vi "LaserControl.vi"() -> ()   [LabVIEW 2015]
uses:
  <vilib>/DAQmx/write.llb/DAQmx Write (Digital Bool 1Line 1Point).vi
  <vilib>/DAQmx/write.llb/DAQmx Write (Analog DBL 1Chan 1Samp).vi
  <vilib>/DAQmx/write.llb/DAQmx Write (Digital 1D Bool NChan 1Samp 1Line).vi
  <vilib>/DAQmx/create/channels.llb/DAQmx Create Channel (DO-Digital Output).vi
  <vilib>/DAQmx/miscellaneous.llb/DAQmx Fill In Error Info.vi
  <vilib>/DAQmx/create/channels.llb/DAQmx Create Channel (AO-Voltage-Basic).vi
panel:
  in  "blueV":dbl
  in  "greenV":dbl
  in  "redV":dbl
  in  "blueAO":dbl(slide) min=0.0 max=5.0 step=0.001 scale=0.0..5.0
  in  "greenAO":dbl(slide) min=0.0 max=5.0 step=0.001 scale=0.0..5.0
  in  "ChangeAOM":bool
  in  "OK Button":bool
  in  "all off":bool
  in  "redAO":dbl(slide) min=0.0 max=5.0 step=0.0001 scale=0.0..5.0
  in  "Green Laser":bool
  in  "Blue Laser":bool
  in  "Red Laser":bool
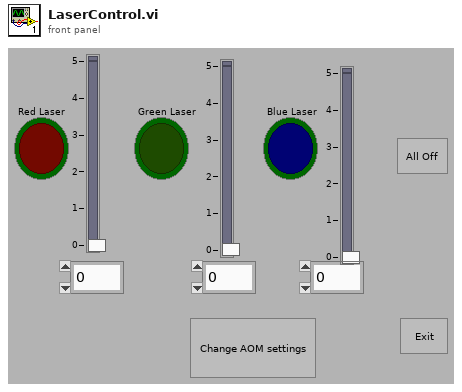
[diagram p1: front panel]
types:
  T1 = typedef "XYZStage.lvlib/XYZStage Configuration.ctl" = cluster{"VISA resource name":refnum<visa-resource-name>, "Timeout (3sec)":u32}
  T2 = cluster{"StageS":i32, "StageL":i32, "currmeas data dir":path, "image OD":u16, "contour OD":u16, "point OD":u16, "AOlines":tag[], "AIlines":tag[], "CI lines":tag[], "DO lines":tag[], "AO names":string[], "CI names":string[], "AI names":string[], "DO names":string[], "CIextensions":string[], "AIextensions":string[], "Voltage to Ygalvo":i32, "Voltage to Xgalvo":i32, "Voltage to patch":i32, "640 shutter":i32, "2P shutter":i32, "LT timestamp":u32, "Vp":i32, "Ip":i32, "camera trigger":i32, "master data dir":path, "voltage to Zpos":i32, "Vto2P":i32, "640 AO":i32, "488 AO":i32, "532 AO":i32, "640TTL":u32, "488TTL":u32, "532TTL":u32, "Device 1 sampleclock out":tag, "Device 1 Starttrigger out":tag, "Device 2 sampleclock in":tag, "Device 2 StartTrigger in ":tag, "2PODTTL":u32, "488 shutter":u32, "LCVR red":u32, "LCVR blue":u32, "Sutter Stage Config":T1}
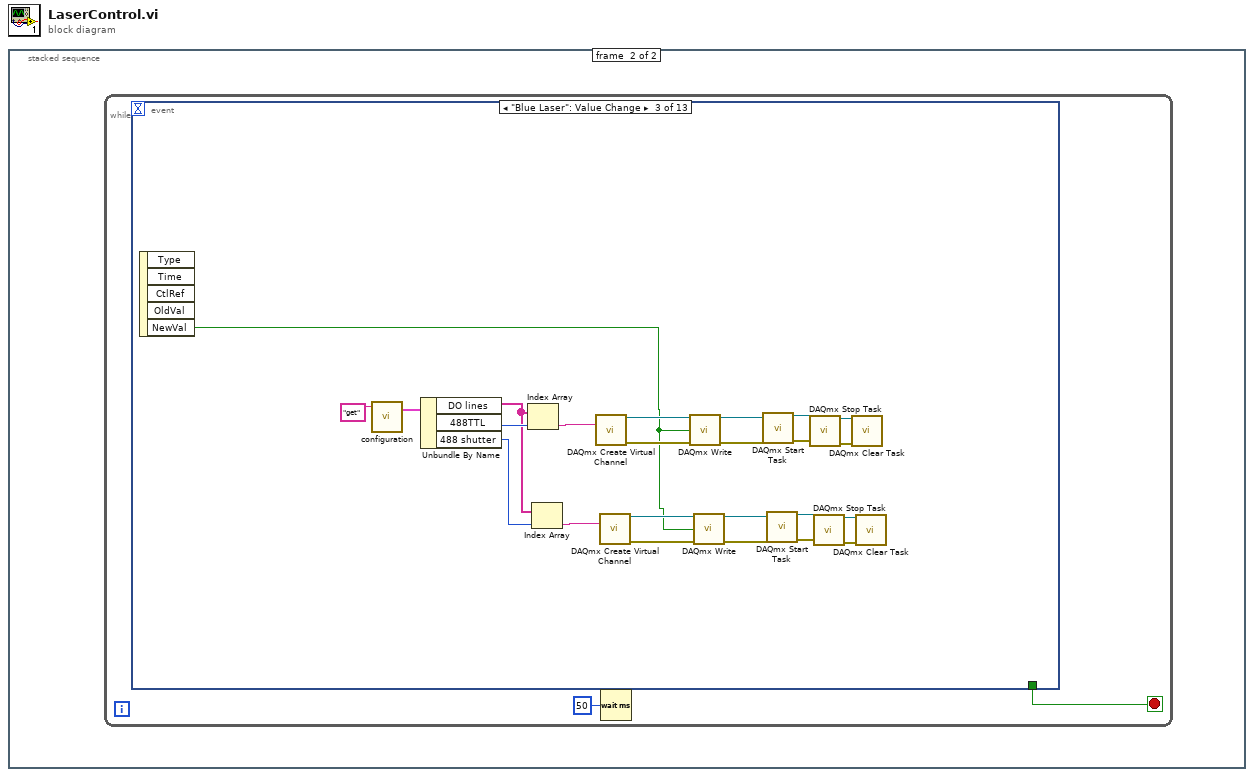
[diagram p0: block diagram]
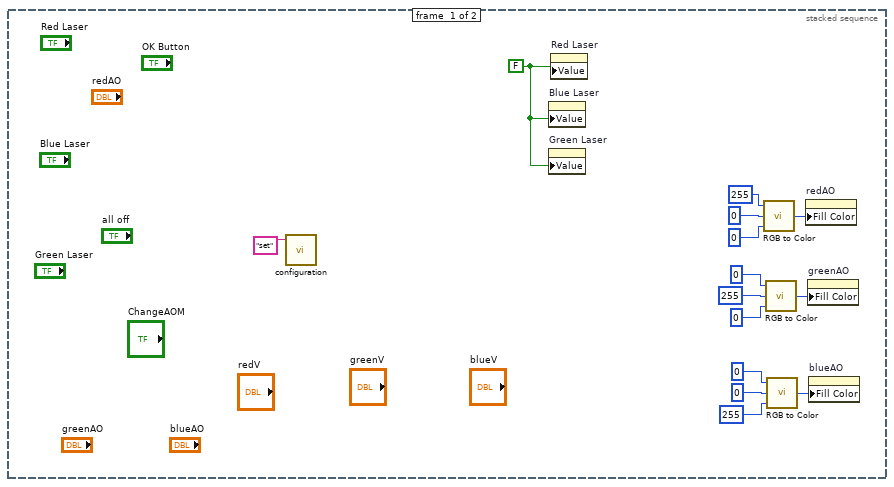
[diagram p2: hidden frame]
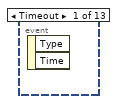
[diagram p3: hidden frame]
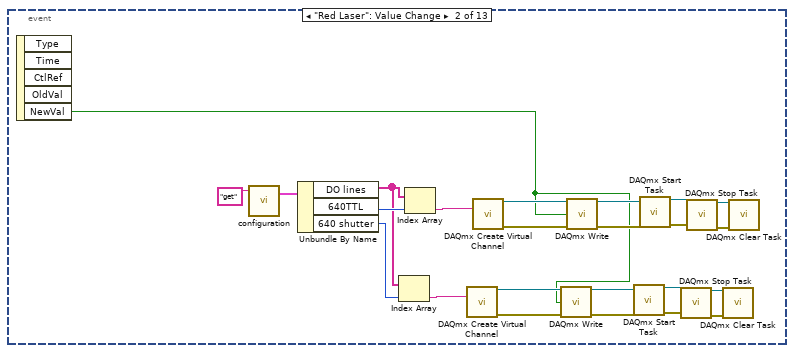
[diagram p4: hidden frame]
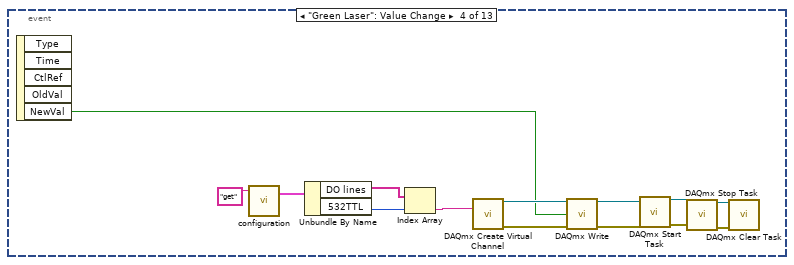
[diagram p5: hidden frame]
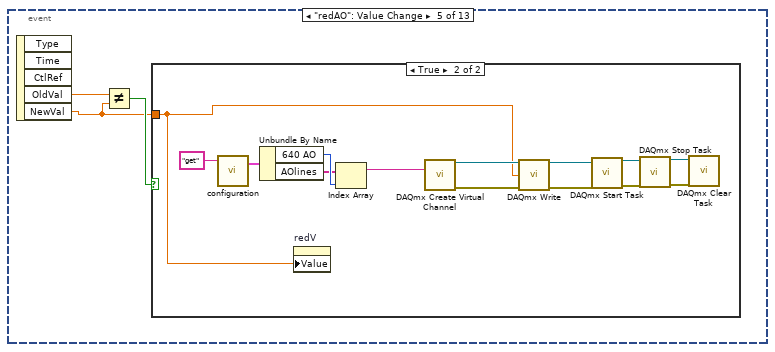
[diagram p6: hidden frame]
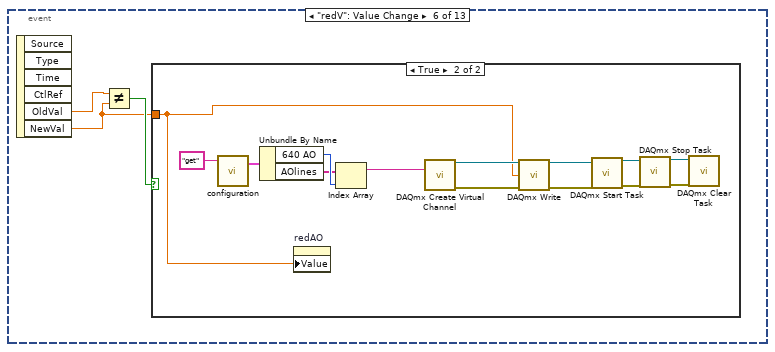
[diagram p8: hidden frame]
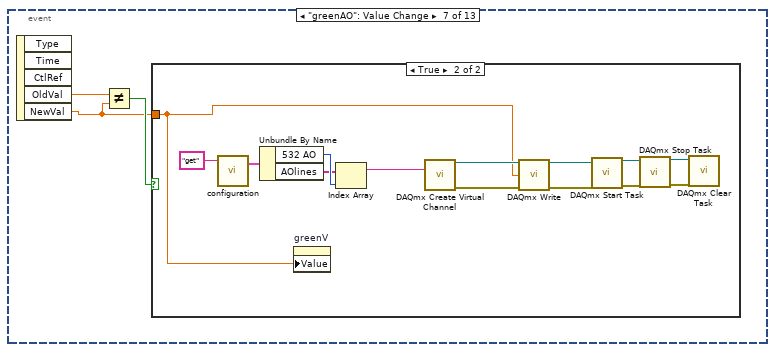
[diagram p10: hidden frame]
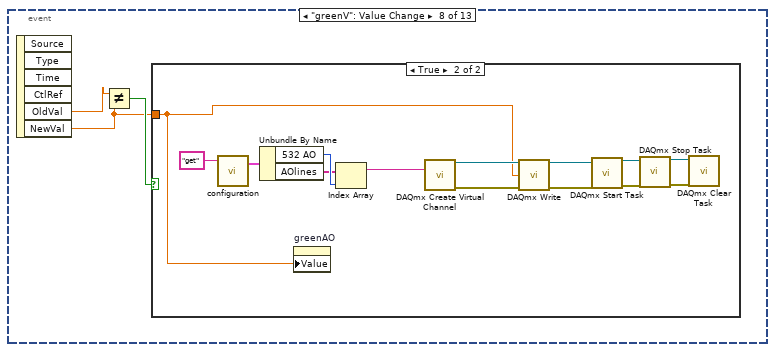
[diagram p12: hidden frame]
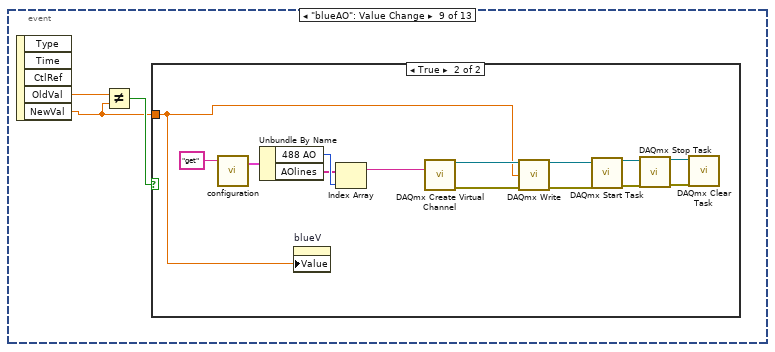
[diagram p14: hidden frame]
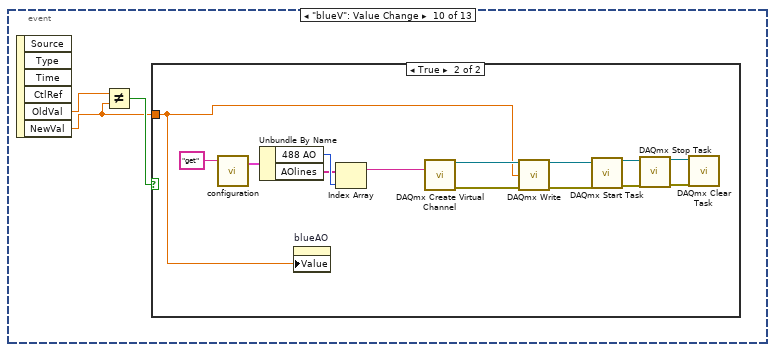
[diagram p16: hidden frame]
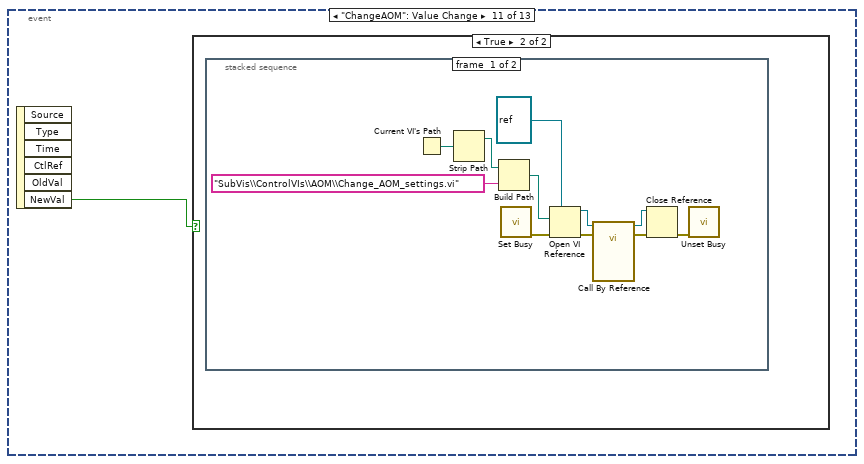
[diagram p18: hidden frame]
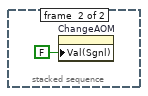
[diagram p20: hidden frame]
diagram:
  n1 = stacked-sequence {
    frame #0 {
      w13 = FALSE
      n2 = call "configuration.vi"("command"="set") -> ()  [unwired: 2 in, 2 out]
      n3 = property on="Blue Laser" class="Bool (strict)"("Value"=w13) -> ()  [unwired: 2 in, 2 out]
      n4 = property on="Green Laser" class="Bool (strict)"("Value"=w13) -> ()  [unwired: 2 in, 2 out]
      n5 = property on="Red Laser" class="Bool (strict)"("Value"=w13) -> ()  [unwired: 2 in, 2 out]
      n6 = call <vilib>:"RGB to Color.vi"("B"=u8 0, "G"=u8 0, "R"=255) -> ("Color"=w14:u32)
      n7 = call <vilib>:"RGB to Color.vi"("B"=u8 0, "G"=u8 255, "R"=0) -> ("Color"=w5:u32)
      n8 = call <vilib>:"RGB to Color.vi"("B"=u8 255, "G"=u8 0, "R"=0) -> ("Color"=w4:u32)
      n9 = property on="redAO" class="Slide (strict)"("Fill Color"=w14) -> ()  [unwired: 2 in, 2 out]
      n10 = property on="greenAO" class="Slide (strict)"("Fill Color"=w5) -> ()  [unwired: 2 in, 2 out]
      n11 = property on="blueAO" class="Slide (strict)"("Fill Color"=w4) -> ()  [unwired: 2 in, 2 out]
    }
    frame #1 {
      n12 = while {
        stop <- w16 stop-if-true
        n13 = event shown="[2] \"Blue Laser\": Value Change" {
          selector: _ -> [_ _ _ _ _ _ _ _ _ _ _ _ _]
          dyn-events: _ -> [_ _ _ _ _ _ _ _ _ _ _ _ _]
          timeout: _ -> [_ _ _ _ _ _ _ _ _ _ _ _ _]
          tunnel: [_ _ _ _ _ _ _ _ _ _ _ _ w220] -> w16
          event Timeout {
            n14 = event-data() -> ()  [unwired: 1 in, 2 out]
          }
          event "Red Laser": Value Change {
            n15 = event-data() -> ("NewVal"=w17:bool)  [unwired: 1 in, 4 out]
            n16 = call "configuration.vi"("command"="get") -> ("config out"=w31:T2)  [unwired: 2 in, 1 out]
            n17 = Unbundle By Name(w31) -> ("DO lines"=w18:tag[], "640TTL"=w30:u32, "640 shutter"=w19:i32)
            n18 = Index Array(array=w18, index=w19) -> (element=w28:tag)
            n19 = Index Array(array=w18, index=w30) -> (element=w29:tag)
            n20 = call-poly <vilib>:"DAQmx Create Virtual Channel.vi"("lines"=w28) -> ("task out"=w26:refnum<k21>, "error out"=w27:errorcluster)  [unwired: 13 in]
            n21 = call-poly <vilib>:"DAQmx Create Virtual Channel.vi"("lines"=w29) -> ("task out"=w34:refnum<k21>, "error out"=w33:errorcluster)  [unwired: 13 in]
            n22 = call-poly <vilib>:"DAQmx Write.vi"("task/channels in"=w26, "data"=w17, "error in"=w27) -> ("task out"=w25:refnum<k21>, "error out"=w24:errorcluster)  [unwired: 10 in, 1 out]
            n23 = call-poly <vilib>:"DAQmx Write.vi"("task/channels in"=w34, "data"=w17, "error in"=w33) -> ("task out"=w35:refnum<k21>, "error out"=w36:errorcluster)  [unwired: 10 in, 1 out]
            n24 = call <vilib>:"DAQmx Start Task.vi"("task/channels in"=w25, "error in"=w24) -> ("task out"=w23:refnum<k21>, "error out"=w22:errorcluster)  [unwired: 12 in]
            n25 = call <vilib>:"DAQmx Start Task.vi"("task/channels in"=w35, "error in"=w36) -> ("task out"=w37:refnum<k21>, "error out"=w38:errorcluster)  [unwired: 12 in]
            n26 = call <vilib>:"DAQmx Stop Task.vi"("task/channels in"=w23, "error in"=w22) -> ("task out"=w21:refnum<k21>, "error out"=w20:errorcluster)  [unwired: 12 in]
            n27 = call <vilib>:"DAQmx Stop Task.vi"("task/channels in"=w37, "error in"=w38) -> ("task out"=w39:refnum<k21>, "error out"=w40:errorcluster)  [unwired: 12 in]
            n28 = call <vilib>:"DAQmx Clear Task.vi"("task in"=w21, "error in"=w20) -> ()  [unwired: 13 in, 1 out]
            n29 = call <vilib>:"DAQmx Clear Task.vi"("task in"=w39, "error in"=w40) -> ()  [unwired: 13 in, 1 out]
          }
          event "Blue Laser": Value Change {
            n30 = event-data() -> ("NewVal"=w43:bool)  [unwired: 1 in, 4 out]
            n31 = call "configuration.vi"("command"="get") -> ("config out"=w55:T2)  [unwired: 2 in, 1 out]
            n32 = Unbundle By Name(w55) -> ("DO lines"=w42:tag[], "488TTL"=w54:u32, "488 shutter"=w41:u32)
            n33 = Index Array(array=w42, index=w54) -> (element=w53:tag)
            n34 = Index Array(array=w42, index=w41) -> (element=w52:tag)
            n35 = call-poly <vilib>:"DAQmx Create Virtual Channel.vi"("lines"=w53) -> ("task out"=w58:refnum<k21>, "error out"=w57:errorcluster)  [unwired: 13 in]
            n36 = call-poly <vilib>:"DAQmx Create Virtual Channel.vi"("lines"=w52) -> ("task out"=w50:refnum<k21>, "error out"=w51:errorcluster)  [unwired: 13 in]
            n37 = call-poly <vilib>:"DAQmx Write.vi"("task/channels in"=w58, "data"=w43, "error in"=w57) -> ("task out"=w59:refnum<k21>, "error out"=w60:errorcluster)  [unwired: 10 in, 1 out]
            n38 = call-poly <vilib>:"DAQmx Write.vi"("task/channels in"=w50, "data"=w43, "error in"=w51) -> ("task out"=w49:refnum<k21>, "error out"=w48:errorcluster)  [unwired: 10 in, 1 out]
            n39 = call <vilib>:"DAQmx Start Task.vi"("task/channels in"=w59, "error in"=w60) -> ("task out"=w61:refnum<k21>, "error out"=w62:errorcluster)  [unwired: 12 in]
            n40 = call <vilib>:"DAQmx Start Task.vi"("task/channels in"=w49, "error in"=w48) -> ("task out"=w47:refnum<k21>, "error out"=w46:errorcluster)  [unwired: 12 in]
            n41 = call <vilib>:"DAQmx Stop Task.vi"("task/channels in"=w61, "error in"=w62) -> ("task out"=w63:refnum<k21>, "error out"=w64:errorcluster)  [unwired: 12 in]
            n42 = call <vilib>:"DAQmx Stop Task.vi"("task/channels in"=w47, "error in"=w46) -> ("task out"=w45:refnum<k21>, "error out"=w44:errorcluster)  [unwired: 12 in]
            n43 = call <vilib>:"DAQmx Clear Task.vi"("task in"=w63, "error in"=w64) -> ()  [unwired: 13 in, 1 out]
            n44 = call <vilib>:"DAQmx Clear Task.vi"("task in"=w45, "error in"=w44) -> ()  [unwired: 13 in, 1 out]
          }
          event "Green Laser": Value Change {
            n45 = event-data() -> ("NewVal"=w70:bool)  [unwired: 1 in, 4 out]
            n46 = call "configuration.vi"("command"="get") -> ("config out"=w68:T2)  [unwired: 2 in, 1 out]
            n47 = Unbundle By Name(w68) -> ("DO lines"=w67:tag[], "532TTL"=w66:u32)
            n48 = Index Array(array=w67, index=w66) -> (element=w65:tag)
            n49 = call-poly <vilib>:"DAQmx Create Virtual Channel.vi"("lines"=w65) -> ("task out"=w72:refnum<k21>, "error out"=w71:errorcluster)  [unwired: 13 in]
            n50 = call-poly <vilib>:"DAQmx Write.vi"("task/channels in"=w72, "data"=w70, "error in"=w71) -> ("task out"=w73:refnum<k21>, "error out"=w74:errorcluster)  [unwired: 10 in, 1 out]
            n51 = call <vilib>:"DAQmx Start Task.vi"("task/channels in"=w73, "error in"=w74) -> ("task out"=w75:refnum<k21>, "error out"=w76:errorcluster)  [unwired: 12 in]
            n52 = call <vilib>:"DAQmx Stop Task.vi"("task/channels in"=w75, "error in"=w76) -> ("task out"=w77:refnum<k21>, "error out"=w78:errorcluster)  [unwired: 12 in]
            n53 = call <vilib>:"DAQmx Clear Task.vi"("task in"=w77, "error in"=w78) -> ()  [unwired: 13 in, 1 out]
          }
          event "redAO": Value Change {
            n54 = event-data() -> ("OldVal"=w80:dbl, "NewVal"=w79:dbl)  [unwired: 1 in, 3 out]
            n55 = Not Equal?(x=w80, y=w79) -> (x != y?=w81:bool)
            n56 = case shown="True" w81 {
              tunnel: w79 -> [_ w82]
              frame False {
              }
              frame True {
                n57 = call "configuration.vi"("command"="get") -> ("config out"=w86:T2)  [unwired: 2 in, 1 out]
                n58 = Unbundle By Name(w86) -> ("640 AO"=w85:i32, "AOlines"=w84:tag[])
                n59 = property on="redV" class="DigNum (strict)"("Value"=w82) -> ()  [unwired: 2 in, 2 out]
                n60 = Index Array(array=w84, index=w85) -> (element=w83:tag)
                n61 = call-poly <vilib>:"DAQmx Create Virtual Channel.vi"("physical channels"=w83) -> ("task out"=w89:refnum<k21>, "error out"=w88:errorcluster)  [unwired: 13 in]
                n62 = call-poly <vilib>:"DAQmx Write.vi"("task/channels in"=w89, "data"=w82, "error in"=w88) -> ("task out"=w90:refnum<k21>, "error out"=w91:errorcluster)  [unwired: 10 in, 1 out]
                n63 = call <vilib>:"DAQmx Start Task.vi"("task/channels in"=w90, "error in"=w91) -> ("task out"=w92:refnum<k21>, "error out"=w93:errorcluster)  [unwired: 12 in]
                n64 = call <vilib>:"DAQmx Stop Task.vi"("task/channels in"=w92, "error in"=w93) -> ("task out"=w94:refnum<k21>, "error out"=w95:errorcluster)  [unwired: 12 in]
                n65 = call <vilib>:"DAQmx Clear Task.vi"("task in"=w94, "error in"=w95) -> ()  [unwired: 13 in, 1 out]
              }
            }
          }
          event "redV": Value Change {
            n66 = event-data() -> ("OldVal"=w97:dbl, "NewVal"=w96:dbl)  [unwired: 1 in, 4 out]
            n67 = Not Equal?(x=w97, y=w96) -> (x != y?=w98:bool)
            n68 = case shown="True" w98 {
              tunnel: w96 -> [_ w99]
              frame False {
              }
              frame True {
                n69 = call "configuration.vi"("command"="get") -> ("config out"=w103:T2)  [unwired: 2 in, 1 out]
                n70 = Unbundle By Name(w103) -> ("640 AO"=w102:i32, "AOlines"=w101:tag[])
                n71 = property on="redAO" class="Slide (strict)"("Value"=w99) -> ()  [unwired: 2 in, 2 out]
                n72 = Index Array(array=w101, index=w102) -> (element=w100:tag)
                n73 = call-poly <vilib>:"DAQmx Create Virtual Channel.vi"("physical channels"=w100) -> ("task out"=w106:refnum<k21>, "error out"=w105:errorcluster)  [unwired: 13 in]
                n74 = call-poly <vilib>:"DAQmx Write.vi"("task/channels in"=w106, "data"=w99, "error in"=w105) -> ("task out"=w107:refnum<k21>, "error out"=w108:errorcluster)  [unwired: 10 in, 1 out]
                n75 = call <vilib>:"DAQmx Start Task.vi"("task/channels in"=w107, "error in"=w108) -> ("task out"=w109:refnum<k21>, "error out"=w110:errorcluster)  [unwired: 12 in]
                n76 = call <vilib>:"DAQmx Stop Task.vi"("task/channels in"=w109, "error in"=w110) -> ("task out"=w111:refnum<k21>, "error out"=w112:errorcluster)  [unwired: 12 in]
                n77 = call <vilib>:"DAQmx Clear Task.vi"("task in"=w111, "error in"=w112) -> ()  [unwired: 13 in, 1 out]
              }
            }
          }
          event "greenAO": Value Change {
            n78 = event-data() -> ("OldVal"=w114:dbl, "NewVal"=w113:dbl)  [unwired: 1 in, 3 out]
            n79 = Not Equal?(x=w114, y=w113) -> (x != y?=w115:bool)
            n80 = case shown="True" w115 {
              tunnel: w113 -> [_ w116]
              frame False {
              }
              frame True {
                n81 = call "configuration.vi"("command"="get") -> ("config out"=w120:T2)  [unwired: 2 in, 1 out]
                n82 = Unbundle By Name(w120) -> ("532 AO"=w119:i32, "AOlines"=w118:tag[])
                n83 = property on="greenV" class="DigNum (strict)"("Value"=w116) -> ()  [unwired: 2 in, 2 out]
                n84 = Index Array(array=w118, index=w119) -> (element=w117:tag)
                n85 = call-poly <vilib>:"DAQmx Create Virtual Channel.vi"("physical channels"=w117) -> ("task out"=w123:refnum<k21>, "error out"=w122:errorcluster)  [unwired: 13 in]
                n86 = call-poly <vilib>:"DAQmx Write.vi"("task/channels in"=w123, "data"=w116, "error in"=w122) -> ("task out"=w124:refnum<k21>, "error out"=w125:errorcluster)  [unwired: 10 in, 1 out]
                n87 = call <vilib>:"DAQmx Start Task.vi"("task/channels in"=w124, "error in"=w125) -> ("task out"=w126:refnum<k21>, "error out"=w127:errorcluster)  [unwired: 12 in]
                n88 = call <vilib>:"DAQmx Stop Task.vi"("task/channels in"=w126, "error in"=w127) -> ("task out"=w128:refnum<k21>, "error out"=w129:errorcluster)  [unwired: 12 in]
                n89 = call <vilib>:"DAQmx Clear Task.vi"("task in"=w128, "error in"=w129) -> ()  [unwired: 13 in, 1 out]
              }
            }
          }
          event "greenV": Value Change {
            n90 = event-data() -> ("OldVal"=w131:dbl, "NewVal"=w130:dbl)  [unwired: 1 in, 4 out]
            n91 = Not Equal?(x=w131, y=w130) -> (x != y?=w132:bool)
            n92 = case shown="True" w132 {
              tunnel: w130 -> [_ w133]
              frame False {
              }
              frame True {
                n93 = call "configuration.vi"("command"="get") -> ("config out"=w137:T2)  [unwired: 2 in, 1 out]
                n94 = Unbundle By Name(w137) -> ("532 AO"=w136:i32, "AOlines"=w135:tag[])
                n95 = property on="greenAO" class="Slide (strict)"("Value"=w133) -> ()  [unwired: 2 in, 2 out]
                n96 = Index Array(array=w135, index=w136) -> (element=w134:tag)
                n97 = call-poly <vilib>:"DAQmx Create Virtual Channel.vi"("physical channels"=w134) -> ("task out"=w140:refnum<k21>, "error out"=w139:errorcluster)  [unwired: 13 in]
                n98 = call-poly <vilib>:"DAQmx Write.vi"("task/channels in"=w140, "data"=w133, "error in"=w139) -> ("task out"=w141:refnum<k21>, "error out"=w142:errorcluster)  [unwired: 10 in, 1 out]
                n99 = call <vilib>:"DAQmx Start Task.vi"("task/channels in"=w141, "error in"=w142) -> ("task out"=w143:refnum<k21>, "error out"=w144:errorcluster)  [unwired: 12 in]
                n100 = call <vilib>:"DAQmx Stop Task.vi"("task/channels in"=w143, "error in"=w144) -> ("task out"=w145:refnum<k21>, "error out"=w146:errorcluster)  [unwired: 12 in]
                n101 = call <vilib>:"DAQmx Clear Task.vi"("task in"=w145, "error in"=w146) -> ()  [unwired: 13 in, 1 out]
              }
            }
          }
          event "blueAO": Value Change {
            n102 = event-data() -> ("OldVal"=w148:dbl, "NewVal"=w147:dbl)  [unwired: 1 in, 3 out]
            n103 = Not Equal?(x=w148, y=w147) -> (x != y?=w149:bool)
            n104 = case shown="True" w149 {
              tunnel: w147 -> [_ w150]
              frame False {
              }
              frame True {
                n105 = call "configuration.vi"("command"="get") -> ("config out"=w154:T2)  [unwired: 2 in, 1 out]
                n106 = Unbundle By Name(w154) -> ("488 AO"=w153:i32, "AOlines"=w152:tag[])
                n107 = property on="blueV" class="DigNum (strict)"("Value"=w150) -> ()  [unwired: 2 in, 2 out]
                n108 = Index Array(array=w152, index=w153) -> (element=w151:tag)
                n109 = call-poly <vilib>:"DAQmx Create Virtual Channel.vi"("physical channels"=w151) -> ("task out"=w157:refnum<k21>, "error out"=w156:errorcluster)  [unwired: 13 in]
                n110 = call-poly <vilib>:"DAQmx Write.vi"("task/channels in"=w157, "data"=w150, "error in"=w156) -> ("task out"=w158:refnum<k21>, "error out"=w159:errorcluster)  [unwired: 10 in, 1 out]
                n111 = call <vilib>:"DAQmx Start Task.vi"("task/channels in"=w158, "error in"=w159) -> ("task out"=w160:refnum<k21>, "error out"=w161:errorcluster)  [unwired: 12 in]
                n112 = call <vilib>:"DAQmx Stop Task.vi"("task/channels in"=w160, "error in"=w161) -> ("task out"=w162:refnum<k21>, "error out"=w163:errorcluster)  [unwired: 12 in]
                n113 = call <vilib>:"DAQmx Clear Task.vi"("task in"=w162, "error in"=w163) -> ()  [unwired: 13 in, 1 out]
              }
            }
          }
          event "blueV": Value Change {
            n114 = event-data() -> ("OldVal"=w164:dbl, "NewVal"=w165:dbl)  [unwired: 1 in, 4 out]
            n115 = Not Equal?(x=w164, y=w165) -> (x != y?=w166:bool)
            n116 = case shown="True" w166 {
              tunnel: w165 -> [_ w167]
              frame False {
              }
              frame True {
                n117 = call "configuration.vi"("command"="get") -> ("config out"=w171:T2)  [unwired: 2 in, 1 out]
                n118 = Unbundle By Name(w171) -> ("488 AO"=w170:i32, "AOlines"=w169:tag[])
                n119 = property on="blueAO" class="Slide (strict)"("Value"=w167) -> ()  [unwired: 2 in, 2 out]
                n120 = Index Array(array=w169, index=w170) -> (element=w168:tag)
                n121 = call-poly <vilib>:"DAQmx Create Virtual Channel.vi"("physical channels"=w168) -> ("task out"=w174:refnum<k21>, "error out"=w173:errorcluster)  [unwired: 13 in]
                n122 = call-poly <vilib>:"DAQmx Write.vi"("task/channels in"=w174, "data"=w167, "error in"=w173) -> ("task out"=w175:refnum<k21>, "error out"=w176:errorcluster)  [unwired: 10 in, 1 out]
                n123 = call <vilib>:"DAQmx Start Task.vi"("task/channels in"=w175, "error in"=w176) -> ("task out"=w177:refnum<k21>, "error out"=w178:errorcluster)  [unwired: 12 in]
                n124 = call <vilib>:"DAQmx Stop Task.vi"("task/channels in"=w177, "error in"=w178) -> ("task out"=w179:refnum<k21>, "error out"=w180:errorcluster)  [unwired: 12 in]
                n125 = call <vilib>:"DAQmx Clear Task.vi"("task in"=w179, "error in"=w180) -> ()  [unwired: 13 in, 1 out]
              }
            }
          }
          event "ChangeAOM": Value Change {
            n126 = event-data() -> ("NewVal"=w181:bool)  [unwired: 1 in, 5 out]
            n127 = case shown="True" w181 {
              frame False {
              }
              frame True {
                n128 = stacked-sequence {
                  frame #0 {
                    n129 = Current VI's Path() -> (path=w183:path)
                    n130 = Strip Path(path=w183) -> (stripped path=w182:path)  [unwired: 1 out]
                    n131 = Build Path(base path=w182, name or relative path="SubVis\\ControlVIs\\AOM\\Change_AOM_settings.vi") -> (appended path=w184:path)
                    n132 = call <vilib>:"Set Busy.vi"() -> ("error out"=w186:errorcluster)  [unwired: 10 in, 1 out]
                    n133 = Open VI Reference(type specifier VI Refnum (for type only)=refnum<vi> refnum, vi path=w184, error in (no error)=w186) -> (vi reference=w188:refnum<vi>, error out=w190:errorcluster)  [unwired: 3 in]
                    n134 = call-by-ref "?"(reference=w188, error in=w190) -> (reference out=w189:refnum<vi>, error out=w191:errorcluster)  [unwired: 11 in, 1 out]
                    n135 = Close Reference(reference=w189, error in (no error)=w191) -> (error out=w187:errorcluster)
                    n136 = call <vilib>:"Unset Busy.vi"("error in (no error)"=w187) -> ()  [unwired: 10 in, 1 out]
                  }
                  frame #1 {
                    n137 = property on="ChangeAOM" class="Bool (strict)"("Val(Sgnl)"=FALSE ("Value (Signaling)")) -> ()  [unwired: 2 in, 2 out]
                  }
                }
              }
            }
          }
          event "all off": Value Change {
            n138 = event-data() -> ("NewVal"=w194:bool)  [unwired: 1 in, 4 out]
            n139 = stacked-sequence {
              tunnel: w194 -> [w195 _]
              frame #0 {
                n140 = case shown="True" w195 {
                  frame False {
                  }
                  frame True {
                    w204 = 0 items=["one channel for each line", "one channel for all lines"] ("line grouping")
                    w206 = FALSE
                    n141 = call "configuration.vi"("command"="get") -> ("config out"=w203:T2)  [unwired: 2 in, 1 out]
                    n142 = Unbundle By Name(w203) -> ("DO lines"=w199:tag[], "640TTL"=w202:u32, "488TTL"=w201:u32, "532TTL"=w200:u32)
                    n143 = property on="Green Laser" class="Bool (strict)"("Value"=w206) -> ()  [unwired: 2 in, 2 out]
                    n144 = property on="Red Laser" class="Bool (strict)"("Value"=w206) -> ()  [unwired: 2 in, 2 out]
                    n145 = property on="Blue Laser" class="Bool (strict)"("Value"=w206) -> ()  [unwired: 2 in, 2 out]
                    n146 = Build Array(w206, w206, w206) -> (w205:bool[])
                    n147 = Build Array(w202, w201, w200) -> (w198:u32[])
                    n148 = for {
                      tunnel: w199 -> [w218]
                      tunnel: w198 -> [w217] mode=indexing
                      tunnel: [w216] -> w197 mode=indexing
                      n149 = Index Array(array=w218, index=w217) -> (element=w216:tag)
                    }
                    n150 = call <vilib>:"DAQmx Flatten Channel String.vi"("names in"=w197) -> ("names out"=w196:string)  [unwired: 13 in, 1 out]
                    n151 = call-poly <vilib>:"DAQmx Create Virtual Channel.vi"("lines"=w196, "line grouping"=w204) -> ("task out"=w209:refnum<k21>, "error out"=w208:errorcluster)  [unwired: 12 in]
                    n152 = call-poly <vilib>:"DAQmx Write.vi"("task/channels in"=w209, "data"=w205, "error in"=w208) -> ("task out"=w210:refnum<k21>, "error out"=w211:errorcluster)  [unwired: 10 in, 1 out]
                    n153 = call <vilib>:"DAQmx Start Task.vi"("task/channels in"=w210, "error in"=w211) -> ("task out"=w212:refnum<k21>, "error out"=w213:errorcluster)  [unwired: 12 in]
                    n154 = call <vilib>:"DAQmx Stop Task.vi"("task/channels in"=w212, "error in"=w213) -> ("task out"=w214:refnum<k21>, "error out"=w215:errorcluster)  [unwired: 12 in]
                    n155 = call <vilib>:"DAQmx Clear Task.vi"("task in"=w214, "error in"=w215) -> ()  [unwired: 13 in, 1 out]
                  }
                }
              }
              frame #1 {
                n156 = property on="all off" class="Bool (strict)"("Value"=FALSE ("all off")) -> ()  [unwired: 2 in, 2 out]
              }
            }
          }
          event "OK Button": Value Change {
            n157 = event-data() -> ("NewVal"=w220:bool)  [unwired: 1 in, 4 out]
          }
        }
        n158 = Wait (ms)(milliseconds to wait=u32 50) -> ()  [unwired: 1 out]
      }
    }
  }
